vi "Camera Image Acquisition.vi"() -> ()   [LabVIEW 2014]
uses:
  Glimpse-master/Microscope plugins/Camera/Glimpse file parameters.ctt
  <vilib>/vision/Image Controls.llb/IMAQ Image.ctl
  SubVIs/Initilize Globals.vi
panel:
  out "Image Size 2":T1 {"V Bin" min=0.0; "H Bin" min=0.0 step=1.0}
  in  "High Capacity?":bool
  out "Continue with acq?":bool
  out "Error Out":errorcluster
  in  "Shutter":i32(ring) items=["Auto", "Stay Open", "Always Closed"]
  out "File properties":T2 {"Max Space Req'd. (Gb)" format="%.2f"}
  in  "Image Type":u32(ring) items=["8 bits", "16 bits", "Float", "Complex", "RGB", "HSL"]
  out "Actual Exposure Time (sec)":dbl
  in  "STOP":bool
  in  "Preview":bool
  in  "Go":bool
  in  "Laser Shutter":T3(radio)
  in  "Number of preview windows":i32=1
  in  "Image Size":T1 {"V Bin" min=0.0; "H Bin" min=0.0 step=1.0}
  in  "Acquisition Parameters":T4={"Readout Mode"=enum."Full Vertical Binning", "Set Acquisition Mode"=enum."(do nothing)", "Trigger Mode"=enum."Internal", "Exposure Time (s)"=0.0, "Accumulation Cycle (s)"=0.0, "Kinetic Cycle Time (s)"=0.0, "Number of Kinetics"=0, "Number of Accumulations"=0, "Set VS Speed"=0, "Pixel Rate"=enum."Standard CCD 3 Mhz 14 bits", "V Shift Amplitude"=enum."+1", "Preamp Gain"=enum."1.0"}
  in  "Set to AOI":bool
  in  "Set to 512 x 300":bool
  in  "Set to Maximum":bool
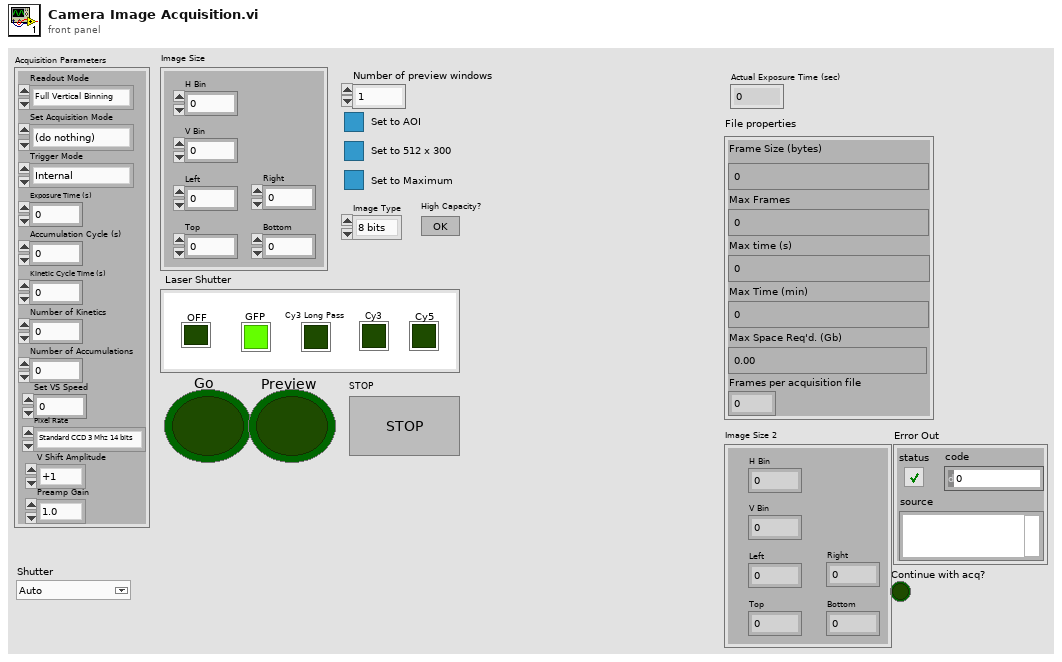
[diagram p1: front panel]
types:
  T1 = cluster{"H Bin":dbl, "V Bin":dbl, "Left":dbl, "Right":dbl, "Top":dbl, "Bottom":dbl}
  T2 = typedef "Glimpse file parameters.ctt" = cluster{"Frame Size (bytes)":u32, "Max Frames":u32, "Max time (s)":u32, "Max Time (min)":u32, "Max Space Req'd. (Gb)":dbl, "Frames per acquisition file":u32}
  T3 = enum32{"GFP", "Cy3 Long Pass", "Cy3", "Cy5", "OFF"}
  T4 = cluster{"Readout Mode":enum16{"Full Vertical Binning", "Multi-Track", "Random-Track", "Single-Track", "Image"}, "Set Acquisition Mode":enum16{"(do nothing)", "Single Scan", "Accumulate", "Kinetics", "Fast Kinetics", "Run till abort"}, "Trigger Mode":enum16{"Internal", "External"}, "Exposure Time (s)":dbl, "Accumulation Cycle (s)":dbl, "Kinetic Cycle Time (s)":dbl, "Number of Kinetics":i32, "Number of Accumulations":i32, "Set VS Speed":i32, "Pixel Rate":enum16{"EM CCD 10 Mhz 14 bits", "EM CCD 5 Mhz 14 bits", "EM CCD 3 Mhz 14 bits", "EM CCD 1 Mhz 16 bits", "Standard CCD 3 Mhz 14 bits", "Standard CCD 1 Mhz 16 bits"}, "V Shift Amplitude":enum16{"normal", "+1", "+2", "+3", "+4"}, "Preamp Gain":enum16{"1.0", "2.4", "5.0"}}
  T5 = typedef "IMAQ Image.ctl" = refnum<image>
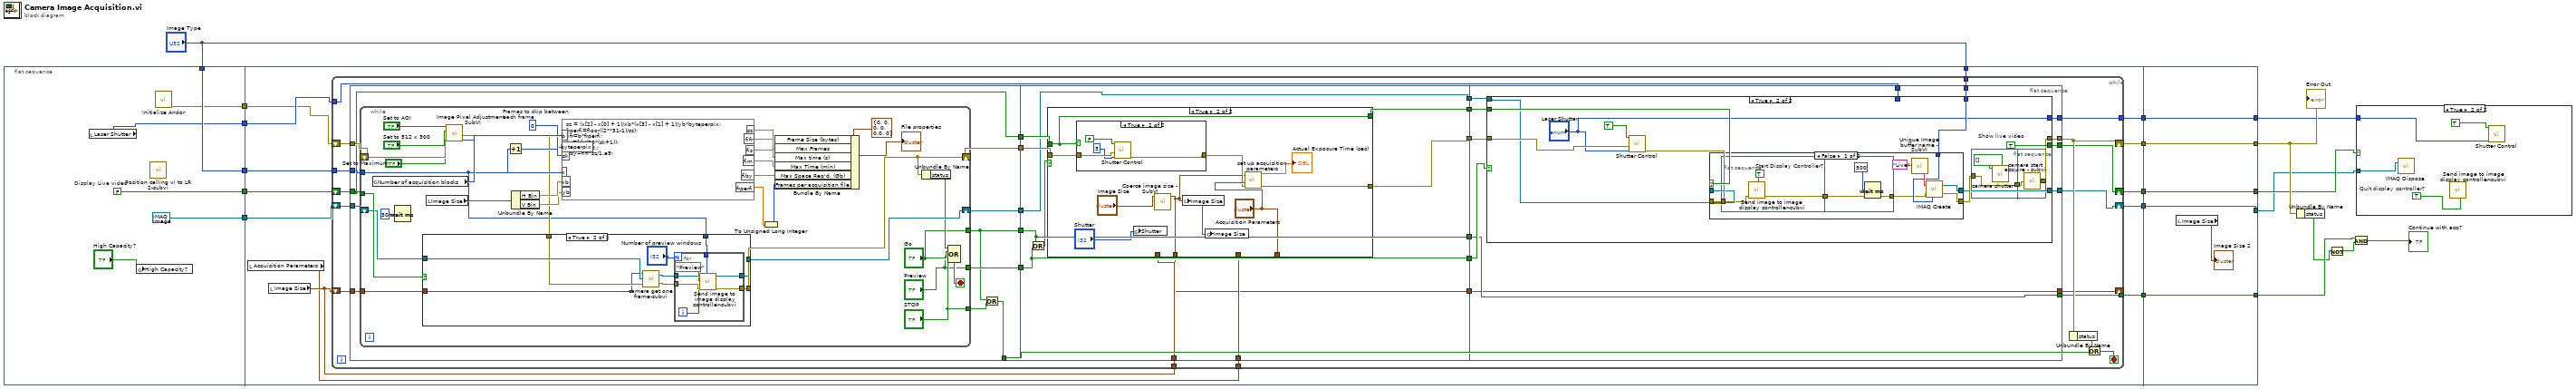
[diagram p0: block diagram]
diagram:
  n1 = flat-sequence {
    tunnel: [w25] -> w19
    tunnel: [w24] -> w18
    tunnel: "Image Type" -> [w24]
    tunnel: [T5 refnum ("New Image")] -> w17
    tunnel: [w22] -> w16
    tunnel: [w21] -> w1
    tunnel: w19 -> [w38]
    tunnel: w18 -> [w37]
    tunnel: w17 -> [w36]
    tunnel: w16 -> [w32]
    tunnel: "Image Type" -> [w33]
    tunnel: [w31] -> w14
    tunnel: [w30] -> w13
    tunnel: [w29] -> w12
    tunnel: [w28] -> w11
    tunnel: [w27] -> w10
    tunnel: w1 -> [w26]
    tunnel: [w211] -> w2
    tunnel: w14 -> [w211]
    tunnel: [w210] -> w9
    tunnel: w13 -> [w210]
    tunnel: [w209] -> w4
    tunnel: w12 -> [w209]
    tunnel: [w208] -> w3
    tunnel: w11 -> [w208]
    tunnel: [w207] -> w8
    tunnel: w10 -> [w207]
    frame #0 {
      w25 = FALSE  # Display Live video
      n2 = local read "Laser Shutter"() -> (w22:T3)
      n3 = global write "Initilize Globals.vi" "High Capacity?"("High Capacity?") -> ()
      n4 = call "Position calling vi to LR 2-subvi.vi"() -> ()  [unwired: 4 in, 2 out]
      n5 = call "Initialize Andor.vi"() -> ("Error Out 2"=w21:errorcluster)  [unwired: 11 in]
    }
    frame #1 {
      n6 = local read "Acquisition Parameters"() -> (w34:T4)
      n7 = local read "Image Size"() -> (w35:T1)
      n8 = while {
        shift-right: [w45] -> w30
        shift-left: w26 -> [w67]
        shift-right: [w44] -> w29
        shift-left: w38 -> [w66]
        tunnel: w37 -> [w65]
        shift-right: [w43] -> w28
        shift-left: w36 -> [w64]
        shift-right: [w41] -> _
        shift-left: w35 -> [w63]
        tunnel: w35 -> [w53]
        tunnel: w34 -> [w52]
        tunnel: w33 -> [w47]
        tunnel: w32 -> [w46]
        tunnel: [w42] -> w31
        tunnel: [w39] -> w27
        stop <- w60 stop-if-true
        n9 = flat-sequence {
          tunnel: w67 -> [w78]
          tunnel: w66 -> [w69]
          tunnel: w65 -> [w77]
          tunnel: w64 -> [w76]
          tunnel: w63 -> [w75]
          tunnel: [w73] -> w62
          tunnel: [w72] -> w61
          tunnel: [w71] -> w59
          tunnel: [w70] -> w57
          tunnel: [w69] -> w56
          tunnel: [w68] -> w51
          tunnel: w62 -> [w139]
          tunnel: w61 -> [w140]
          tunnel: w57 -> [w134]
          tunnel: w56 -> [w137]
          tunnel: [w140] -> w55
          tunnel: [w139] -> w54
          tunnel: w53 -> [w136]
          tunnel: w52 -> [w135]
          tunnel: w51 -> [w133]
          tunnel: [w133] -> w50
          tunnel: [w132] -> w49
          tunnel: [w131] -> w48
          tunnel: [w130] -> w40
          tunnel: w55 -> [w169]
          tunnel: w54 -> [w170]
          tunnel: w50 -> [w168]
          tunnel: [w169] -> w39
          tunnel: w49 -> [w167]
          tunnel: w48 -> [w166]
          tunnel: w47 -> [w165]
          tunnel: w46 -> [w164]
          tunnel: [w163] -> w45
          tunnel: [w162] -> w44
          tunnel: [w161] -> w43
          tunnel: [w160] -> w42
          tunnel: [w159] -> w41
          tunnel: w40 -> [w159]
          frame #0 {
            n10 = while {
              shift-right: [w85] -> w70
              shift-left: w78 -> [w110]
              tunnel: w69 -> [w90]
              tunnel: w77 -> [w86]
              shift-right: [w84] -> w68
              shift-left: w76 -> [w89]
              tunnel: w75 -> [w88]
              tunnel: ["STOP"] -> w74
              tunnel: ["Go"] -> w72
              tunnel: ["Preview"] -> w73
              stop <- w82 stop-if-true
              w101 = u16 0  # Frames to skip between each frame
              n11 = global read "Initilize Globals.vi" "Number of acquisition blocks"() -> (w106:i8)
              n12 = Wait (ms)(milliseconds to wait=u32 30) -> ()  [unwired: 1 out]
              n13 = local read "Image Size"() -> (w104:T1)
              n14 = call "Image Pixel Adjustment - SubVI.vi"("error in"=w110, "Set to Maximum"="Set to Maximum", "Set to 512 x 300"="Set to 512 x 300", "Set to AOI"="Set to AOI") -> ("Pixels Out"=w105:i32[], "Error Out (no error)"=w87:errorcluster)  [unwired: 6 in]
              n15 = case shown="True" w90 {
                tunnel: w89 -> [w113 w122]
                tunnel: [w113 w116] -> w84
                tunnel: w88 -> [_ w114]
                tunnel: w87 -> [w112 w121]
                tunnel: w86 -> [_ w117]
                tunnel: [w112 w115] -> w85
                frame False {
                }
                frame True {
                  n16 = call "camera get one frame-subvi.vi"("error in"=w121, "New Image"=w122, "Image Size"=w114) -> ("error out"=w118:errorcluster, "Image Out"=w119:T5)
                  n17 = for {
                    N: "Number of preview windows" -> [_]
                    tunnel: w119 -> [w127]
                    tunnel: w118 -> [w128]
                    tunnel: w117 -> [w129]
                    tunnel: [w124] -> w116
                    tunnel: [w123] -> w115
                    i -> [w125]
                    n18 = call "Send image to image display controller-subvi.vi"("Image"=w127, "Window Title"="Preview" ("Window Title\n(Window only)"), "Window Number"=w125, "error in"=w128, "Image Type"=w129) -> ("Image Out"=w124:T5, "error out"=w123:errorcluster)  [unwired: 4 in]
                  }
                }
              }
              n19 = Increment(x=w86) -> (x+1=w100:u32)
              n20 = Unbundle By Name(w104) -> ("H Bin"=w103:dbl, "V Bin"=w102:dbl)
              n21 = formula code="sz = (x[2] - x[0] + 1)/xb*(x[3] - x[1] + 1)/yb*byteperpix;\nfrperfi=floor((2**31-1)/sz);\nfifr=b*frperfi;\nfis=fifr/(30*(sk+1));\nfim=fis/60.;\nfiby=fifr*sz/1.e9;"("x"=w105, "b"=w106, "sk"=w101, "xb"=w103, "yb"=w102, "byteperpix"=w100) -> ("sz"=w93:dbl, "fifr"=w94:dbl, "fis"=w95:dbl, "fim"=w96:dbl, "fiby"=w97:dbl, "frperfi"=w99:dbl)
              n22 = To Unsigned Long Integer(number=w99) -> (unsigned 32bit integer=w98:u32)
              n23 = Bundle By Name(cluster=T2 {"Frame Size (bytes)"=0, "Max Frames"=0, "Max time (s)"=0, "Max Time (min)"=0, "Max Space Req'd. (Gb)"=0.0, "Frames per acquisition file"=0} ("Glimpse file properties"), "Frame Size (bytes)"=w93, "Max Frames"=w94, "Max time (s)"=w95, "Max Time (min)"=w96, "Max Space Req'd. (Gb)"=w97, "Frames per acquisition file"=w98) -> (→"File properties":T2)
              n24 = Unbundle By Name(w85) -> ("status"=w83:bool)
              n25 = Compound Arithmetic op=OR(w83, "Go", "Preview", "STOP") -> (w82:bool)
            }
            n26 = Or(x=w72, y=w74) -> (x .or. y?=w71:bool)
          }
          frame #1 {
            n27 = Or(x=w140, y=w139) -> (x .or. y?=w138:bool)
            n28 = case shown="True" w138 {
              tunnel: w137 -> [w144 w153]
              tunnel: [w144 w153] -> w131
              tunnel: [w142 "Acquisition Parameters"] -> _
              tunnel: [w143 w145] -> w130
              tunnel: w136 -> [w143 _]
              tunnel: w135 -> [w142 _]
              tunnel: w134 -> [w141 w149]
              tunnel: [w141 w146] -> w132
              frame False {
              }
              frame True {
                n29 = case shown="True" w153 {
                  tunnel: w149 -> [w154 w158]
                  tunnel: [w154 w156] -> w148
                  frame False {
                  }
                  frame True {
                    n30 = call "Shutter Control.vi"("Laser Shutter"=3, "error in"=w158, "Camera Shutter"=FALSE) -> ("error out"=w156:errorcluster)  [unwired: 8 in]
                  }
                }
                n31 = global write "Initilize Globals.vi" "Shutter"("Shutter") -> ()
                n32 = call "Coerce image size - SubVI.vi"("Image Size"="Image Size") -> ("Image Size 2"=w145:T1)  [unwired: 10 in]
                n33 = local write "Image Size"(w145) -> ()
                n34 = global write "Initilize Globals.vi" "Image Size"(w145) -> ()
                n35 = call "set up acquisition parameters.vi"("error in (no error)"=w148, "Acquisition Parameters"="Acquisition Parameters", "Image Size"=w145) -> ("error out"=w146:errorcluster, "Exposure"=→"Actual Exposure Time (sec)":dbl)  [unwired: 3 in, 2 out]
              }
            }
          }
          frame #2 {
            n36 = case shown="True" w170 {
              tunnel: w168 -> [w171 w182]
              tunnel: w167 -> [w174 w185]
              tunnel: w166 -> [w172 w186]
              tunnel: [w174 w176] -> w163
              tunnel: w165 -> [_ w181]
              tunnel: [w172 w180] -> w162
              tunnel: [w173 "Laser Shutter"] -> w160
              tunnel: w164 -> [w173 _]
              tunnel: [w171 w175] -> w161
              frame False {
              }
              frame True {
                w180 = TRUE  # Show live video
                n37 = call "Shutter Control.vi"("Laser Shutter"="Laser Shutter", "error in"=w185, "Camera Shutter"=TRUE) -> ("error out"=w183:errorcluster)  [unwired: 8 in]
                n38 = case shown="False" w186 {
                  tunnel: w183 -> [w198 w204]
                  tunnel: w182 -> [_ w205]
                  tunnel: [w195 w205] -> w175
                  tunnel: [w196 w204] -> w178
                  tunnel: w181 -> [w192 _]
                  frame False {
                    n39 = flat-sequence {
                      tunnel: w198 -> [w201]
                      tunnel: [w199] -> w197
                      tunnel: [w203] -> w191
                      tunnel: w197 -> [w203]
                      frame #0 {
                        w200 = TRUE  # Start Display Controller?
                        n40 = call "Send image to image display controller-subvi.vi"("error in"=w201, "Start display controller?"=w200) -> ("error out"=w199:errorcluster)  [unwired: 7 in, 1 out]
                      }
                      frame #1 {
                        n41 = Wait (ms)(milliseconds to wait=u32 500) -> ()  [unwired: 1 out]
                      }
                    }
                    n42 = call "Unique Image buffer name - SubVI.vi"("Buffer  base name"="Live") -> ("Image Name"=w194:string)  [unwired: 1 in]
                    n43 = call "IMAQ Create"("Image Name"=w194, "Image Type"=w192, "error in (no error)"=w191) -> ("New Image"=w195:T5, "error out"=w196:errorcluster)  [unwired: 1 in, 1 out]
                  }
                  frame True {
                  }
                }
                n44 = flat-sequence {
                  tunnel: w178 -> [w188]
                  tunnel: [w188] -> w177
                  tunnel: w177 -> [w190]
                  tunnel: [w189] -> w176
                  frame #0 {
                    n45 = call "camera shutter.vi"("Array"=bool[] []) -> ()  [unwired: 10 in, 1 out]
                  }
                  frame #1 {
                    n46 = call "camera start acquire - subvi.vi"("error in"=w190) -> ("error out"=w189:errorcluster)
                  }
                }
              }
            }
          }
        }
        n47 = Unbundle By Name(w45) -> ("status"=w58:bool)
        n48 = Or(x=w58, y=w59) -> (x .or. y?=w60:bool)
      }
    }
    frame #2 {
      n49 = local read "Image Size"() -> (→"Image Size 2":T1)
    }
  }
  n50 = Unbundle By Name(w9) -> ("status"=w7:bool)
  n51 = Not(x=w7) -> (.not. x?=w6:bool)
  n52 = And(x=w8, y=w6) -> (x .and. y?=→"Continue with acq?":bool)
  n53 = case shown="True" w4 {
    tunnel: w3 -> [_ w214]
    tunnel: w2 -> [_ w213]
    frame False {
    }
    frame True {
      w215 = TRUE  # Quit display controller?
      n54 = call "IMAQ Dispose"("Image"=w214) -> ()  [unwired: 2 in, 4 out]
      n55 = call "Send image to image display controller-subvi.vi"("Quit display controller?"=w215) -> ()  [unwired: 8 in, 2 out]
      n56 = call "Shutter Control.vi"("Laser Shutter"=w213, "Camera Shutter"=TRUE) -> ()  [unwired: 9 in, 1 out]
    }
  }
  "Error Out" <- w9
